vi "Scopes.vi"(11 "Request in":refnum<class "Request.lvclass">) -> (2 "Scopes":string[](array[string]))   [LabVIEW 2020, in "OAuth2.lvlib" / "Request.lvclass"]
uses:
  Request.lvclass
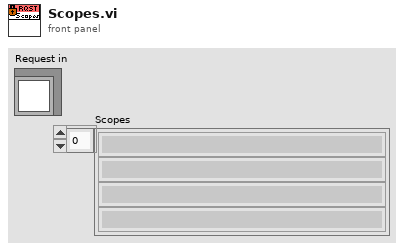
[diagram p1: front panel]
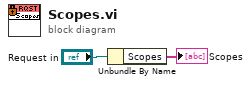
[diagram p0: block diagram]
diagram:
  n1 = Unbundle By Name("Request in") -> ("Scopes"=→"Scopes":string[])
